vi "Write Customer Name.vi"(10 "Customer Name":string, 11 "Abstract Beverage in":refnum<class "Abstract Beverage.lvclass">) -> (3 "Abstract Beverage in 2":refnum<class "Abstract Beverage.lvclass">)   [LabVIEW 2013, in "Abstract Beverage.lvclass"]
uses:
  Abstract Beverage.lvclass
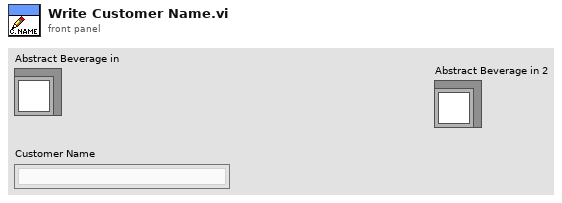
[diagram p1: front panel]
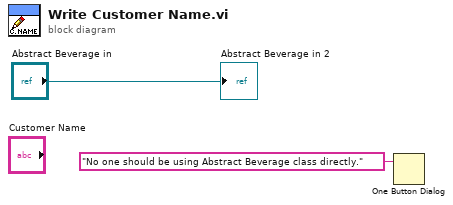
[diagram p0: block diagram]
diagram:
  n1 = One Button Dialog(message="No one should be using Abstract Beverage class directly.") -> ()  [unwired: 1 in, 1 out]
  "Abstract Beverage in 2" <- "Abstract Beverage in"
